vi "RD Enum Device Info.vi"(7 "handle":u64, 8 "error in (no error)":errorcluster caption="错误输入（无错误）", 9 "SerialNumber":string, 10 "Description":string, 11 "i":i32) -> (0 "error out":errorcluster caption="错误输出", 1 "SerialNumber out":string, 2 "Description out":string, 3 "function return":i32, 5 "handle out":u64)   [LabVIEW 2018, in "InstrumentsPlayground.lvlib"]
doc: "CLIFFAPI int CliffEnumDeviceInfo (int i, char* Description,char* SerialNumber,FT_HANDLE *handle);"
uses:
  InstrumentsPlayground.lvlib
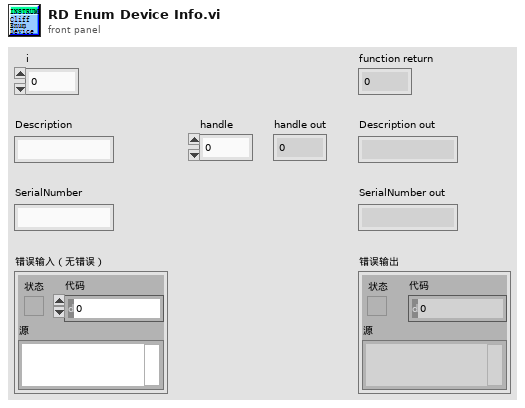
[diagram p1: front panel]
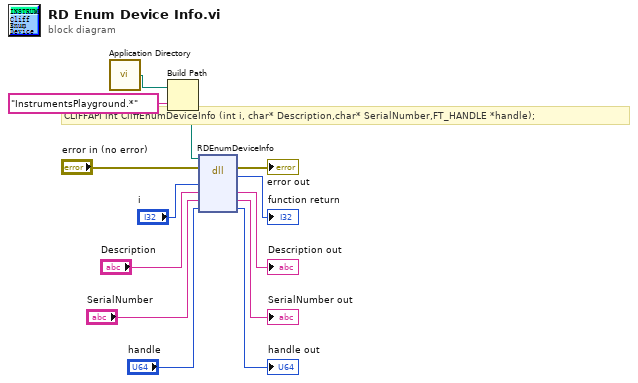
[diagram p0: block diagram]
diagram:
  # "CLIFFAPI int CliffEnumDeviceInfo (int i, char* Description,char* SerialNumber,FT_HANDLE *handle);"
  n1 = call <vilib>:"Application Directory.vi"() -> ("Application Directory"=w2:path)
  n2 = Build Path(base path=w2, name or relative path="InstrumentsPlayground.*" ("名称或相对路径")) -> (appended path=w1:path)
  n3 = dll-call lib="E:/work/YZCourse_Xtext/Cliff/API/LabVIEW lib/InstrumentsPlayground.*" fn="RDEnumDeviceInfo"(path in=w1, error in="error in (no error)", "i"="i", "Description"="Description", "SerialNumber"="SerialNumber", "handle"="handle") -> (error out=→"error out":errorcluster, "返回类型"=→"function return":i32, "Description"=→"Description out":string, "SerialNumber"=→"SerialNumber out":string, "handle"=→"handle out":u64)  [unwired: 2 in, 1 out]
